vi "SetZeroFCG.vi"(8 "error in (no error)":errorcluster) -> (0 "error out":errorcluster)   [LabVIEW 2011]
uses:
  Variables/GlobalSetGetConfigureCamera.vi
  Variables/ccdChipPixels.vi
  Variables/GlobalSetGetHeidenhainParameters.vi
  Variables/GlobalSetNumberOfDigits_PhysikalInstruments.vi
  Variables/GrapRoi.vi
  Variables/GlobalGetPhysikalInstrumentsOnOff.vi
  Variables/StartStopMesaurement.vi
  Variables/GlobalGetMesaurementStatus.vi
  Variables/GlobalLaserEmissionOnOffInterlook.vi
  Variables/GlobalGetHeidenhainDriftOnOff.vi
  Variables/GlobalGetConfigurationStatus.vi
  Variables/GlobalGetInitialisationStatus.vi
  Variables/GlobalGetKoherasLaserOnOff.vi
  Variables/GlobalGetAOTFOnOff.vi
  Variables/GlobalGetAvantesSpectrometerOnOff.vi
  Variables/GlobalGetCamerasOnOff.vi
  Variables/SetRoi.vi
  Variables/GetPicture.vi
  Variables/StopGetPic.vi
  Variables/GlobalSetGetParametersAvantes.vi
  Variables/GlobalSetGetPositionParameters.vi
  Variables/GlobalSetGetTriggerForPointMeasurement.vi
  Variables/GlobalSetGetPixelOfRoi.vi
  Variables/GetSetGlobalPath2StoreStackData.vi
  Variables/cameraHandler.vi
  Variables/GlobalCameraDebugTemperature.vi
  Variables/ScannerMirrorStatus.vi
  Variables/GlobalGetSetMeasurementType.vi
  Variables/GlobalSetNumberOfDigits_Scanners.vi
  Variables/GlobalImage.vi
panel:
  in  "out":T1
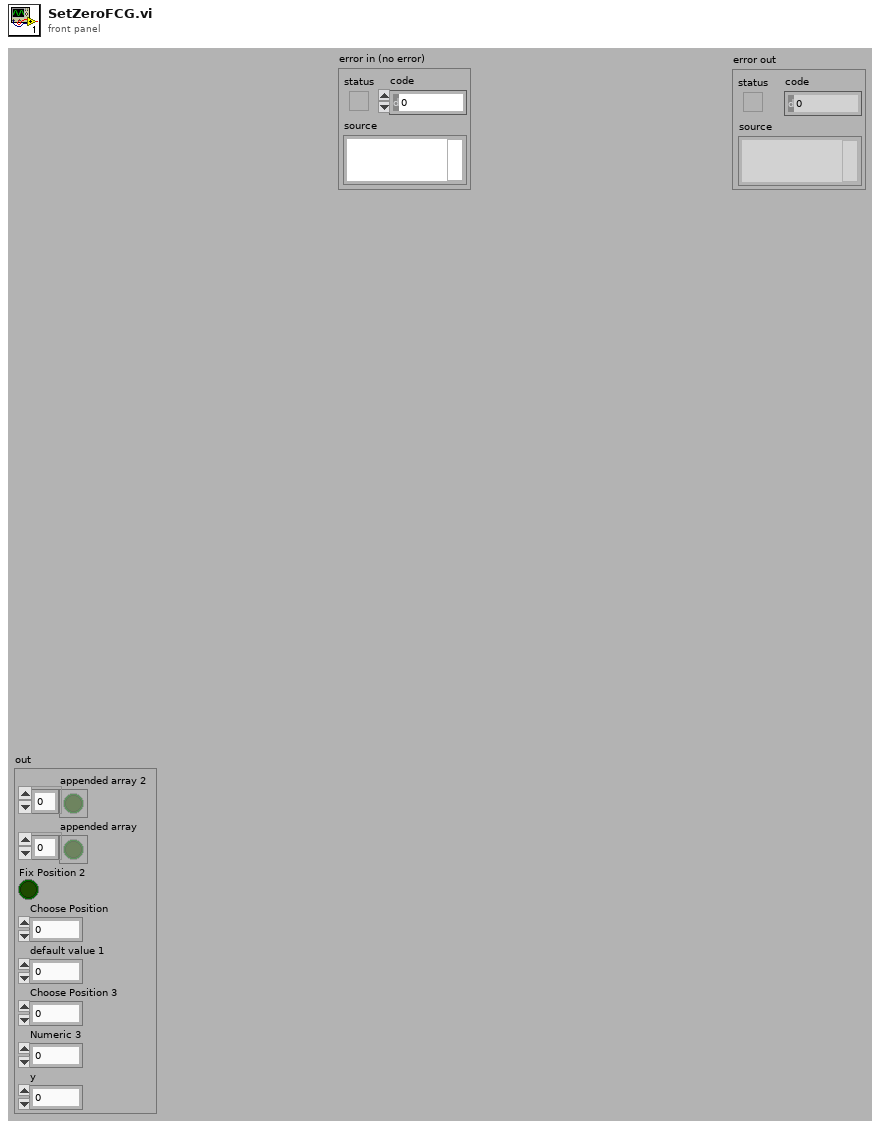
[diagram p1: front panel]
types:
  T1 = cluster{"appended array 2":bool[], "appended array":bool[], "Fix Position 2":bool, "Choose Position":dbl, "default value 1":dbl, "Choose Position 3":dbl, "Numeric 3":i32, "y":i32}
  T2 = cluster{"numbers of \nmeasurements":i16, "startPixel":u16, "stopPixel":u16, "intTime / [ms]":sgl, "backgroundSubtract":bool, "numAvg":u32}
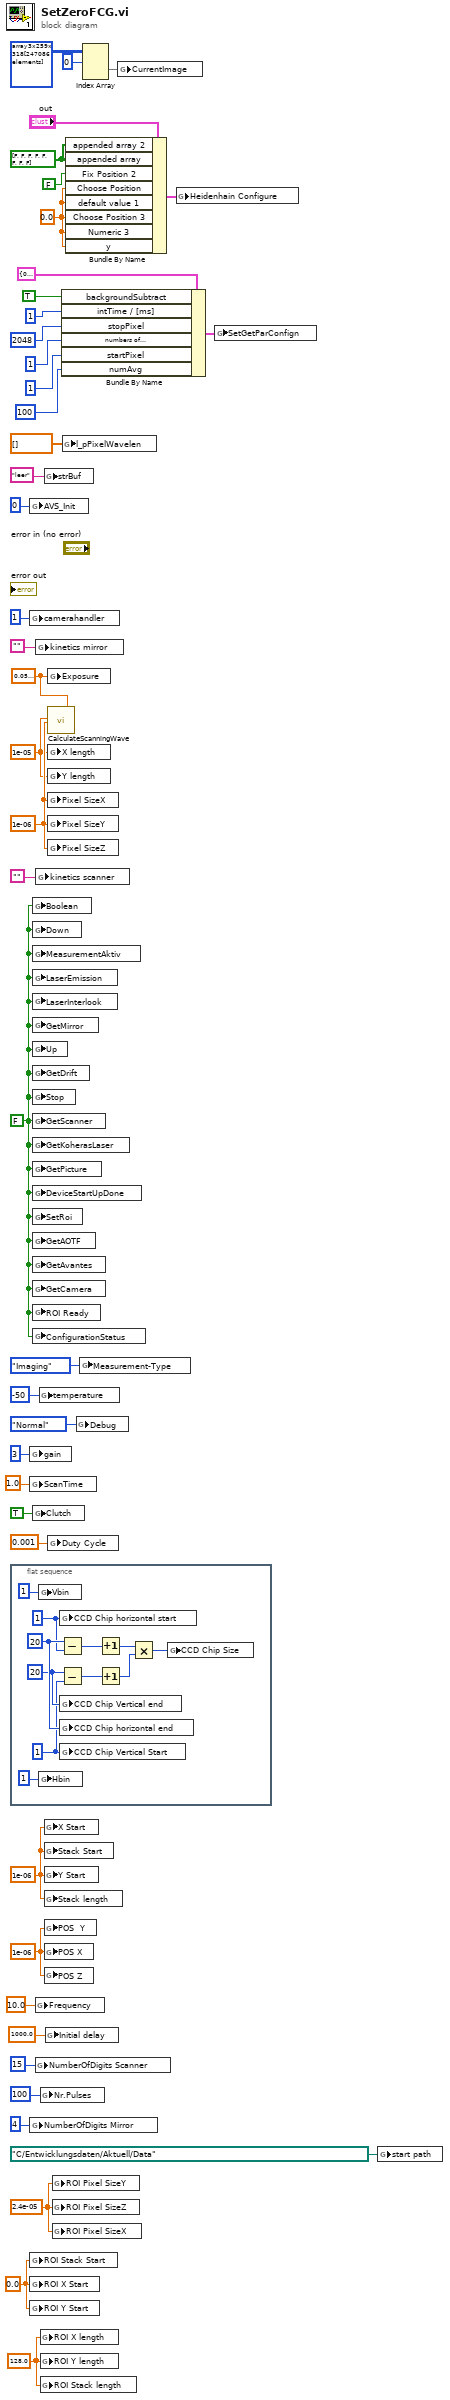
[diagram p0: block diagram]
diagram:
  w18 = 128.0 ("ROI Stack length")
  w19 = 0.0 ("ROI Stack Start")
  w20 = 2.4e-05 ("ROI Pixel SizeX")
  w14 = 1e-05 ("X length")
  w17 = 1e-06 ("X Start")
  w15 = 1e-06 ("Pixel SizeX")
  w29 = 1e-06 ("Duty Cycle")
  w1 = FALSE ("andor 2")
  w16 = sgl 0.05 ("ExpTime")
  w42 = 0.0 ("Choose Position")
  w43 = bool[] [FALSE, FALSE, FALSE, FALSE, FALSE, FALSE, FALSE, FALSE] ("appended array")
  n1 = flat-sequence {
    frame #0 {
      w48 = 20 ("CCD Chip Vertical end")
      w46 = 1 ("CCD Chip Vertical Start")
      w47 = 20 ("CCD Chip horizontal end")
      w45 = 1
      n2 = global write "GlobalSetGetConfigureCamera.vi" "Vbin"(1 ("Vbin")) -> ()
      n3 = global write "GlobalSetGetConfigureCamera.vi" "Hbin"(1 ("Hbin")) -> ()
      n4 = Subtract(x=w48, y=w45) -> (x-y=w50:i32)
      n5 = Subtract(x=w47, y=w46) -> (x-y=w49:i32)
      n6 = global write "ccdChipPixels.vi" "CCD Chip horizontal start"(w45) -> ()
      n7 = global write "ccdChipPixels.vi" "CCD Chip Vertical end"(w47) -> ()
      n8 = global write "ccdChipPixels.vi" "CCD Chip horizontal end"(w48) -> ()
      n9 = global write "ccdChipPixels.vi" "CCD Chip Vertical Start"(w46) -> ()
      n10 = Increment(x=w50) -> (x+1=w52:i32)
      n11 = Increment(x=w49) -> (x+1=w51:i32)
      n12 = Multiply(x=w52, y=w51) -> (x*y=w55:i32)
      n13 = global write "ccdChipPixels.vi" "CCD Chip Size"(w55) -> ()
    }
  }
  n14 = global write "GlobalSetGetParametersAvantes.vi" "AVS_Init"(0 ("AVS_Init")) -> ()
  n15 = global write "cameraHandler.vi" "camerahandler"(1 ("camerahandler")) -> ()
  n16 = global write "GlobalSetGetConfigureCamera.vi" "gain"(3 ("gain")) -> ()
  n17 = global write "GlobalSetGetPositionParameters.vi" "ScanTime"(1.0 ("Duty Cycle")) -> ()
  n18 = global write "GlobalSetNumberOfDigits_PhysikalInstruments.vi" "NumberOfDigits Mirror"(4 ("NumberOfDigits")) -> ()
  n19 = global write "GlobalSetGetPixelOfRoi.vi" "ROI Stack Start"(w19) -> ()
  n20 = global write "GlobalSetGetPixelOfRoi.vi" "ROI X Start"(w19) -> ()
  n21 = global write "GlobalSetGetPixelOfRoi.vi" "ROI Y Start"(w19) -> ()
  n22 = global write "StartStopMesaurement.vi" "Boolean"(w1) -> ()
  n23 = global write "GlobalSetGetHeidenhainParameters.vi" "Down"(w1) -> ()
  n24 = global write "GlobalGetMesaurementStatus.vi" "MeasurementAktiv"(w1) -> ()
  n25 = global write "GlobalLaserEmissionOnOffInterlook.vi" "LaserEmission"(w1) -> ()
  n26 = global write "GlobalLaserEmissionOnOffInterlook.vi" "LaserInterlook"(w1) -> ()
  n27 = global write "GlobalGetPhysikalInstrumentsOnOff.vi" "GetMirror"(w1) -> ()
  n28 = global write "GlobalSetGetHeidenhainParameters.vi" "Up"(w1) -> ()
  n29 = global write "GlobalGetHeidenhainDriftOnOff.vi" "GetDrift"(w1) -> ()
  n30 = global write "StopGetPic.vi" "Stop"(w1) -> ()
  n31 = global write "GlobalGetPhysikalInstrumentsOnOff.vi" "GetScanner"(w1) -> ()
  n32 = global write "GlobalGetKoherasLaserOnOff.vi" "GetKoherasLaser"(w1) -> ()
  n33 = global write "GetPicture.vi" "GetPicture"(w1) -> ()
  n34 = global write "GlobalGetInitialisationStatus.vi" "DeviceStartUpDone"(w1) -> ()
  n35 = global write "SetRoi.vi" "SetRoi"(w1) -> ()
  n36 = global write "GlobalGetAOTFOnOff.vi" "GetAOTF"(w1) -> ()
  n37 = global write "GlobalGetAvantesSpectrometerOnOff.vi" "GetAvantes"(w1) -> ()
  n38 = global write "GlobalGetCamerasOnOff.vi" "GetCamera"(w1) -> ()
  n39 = global write "GrapRoi.vi" "ROI Ready"(w1) -> ()
  n40 = global write "GlobalGetConfigurationStatus.vi" "ConfigurationStatus"(w1) -> ()
  n41 = global write "GlobalSetGetHeidenhainParameters.vi" "Clutch"(TRUE ("Clutch")) -> ()
  n42 = global write "GlobalSetGetTriggerForPointMeasurement.vi" "Frequency"(10.0 ("Frequency")) -> ()
  n43 = global write "GlobalSetNumberOfDigits_Scanners.vi" "NumberOfDigits Scanner"(15 ("NumberOfDigits Scanner")) -> ()
  n44 = global write "ScannerMirrorStatus.vi" "kinetics mirror"("") -> ()
  n45 = global write "ScannerMirrorStatus.vi" "kinetics scanner"("") -> ()
  n46 = global write "GlobalCameraDebugTemperature.vi" "temperature"(-50 ("temperature")) -> ()
  n47 = global write "GlobalSetGetTriggerForPointMeasurement.vi" "Nr.Pulses"(100 ("Nr.Pulses")) -> ()
  n48 = global write "GlobalSetGetPixelOfRoi.vi" "ROI X length"(w18) -> ()
  n49 = global write "GlobalSetGetPixelOfRoi.vi" "ROI Y length"(w18) -> ()
  n50 = global write "GlobalSetGetPixelOfRoi.vi" "ROI Stack length"(w18) -> ()
  n51 = global write "GlobalSetGetParametersAvantes.vi" "strBuf"("leer" ("strBuf")) -> ()
  n52 = global write "GlobalSetGetPixelOfRoi.vi" "X Start"(w17) -> ()
  n53 = global write "GlobalSetGetPixelOfRoi.vi" "Stack Start"(w17) -> ()
  n54 = global write "GlobalSetGetPixelOfRoi.vi" "Y Start"(w17) -> ()
  n55 = global write "GlobalSetGetPixelOfRoi.vi" "Stack length"(w17) -> ()
  n56 = global write "GlobalSetGetPositionParameters.vi" "POS  Y"(w29) -> ()
  n57 = global write "GlobalSetGetPositionParameters.vi" "POS X"(w29) -> ()
  n58 = global write "GlobalSetGetPositionParameters.vi" "POS Z"(w29) -> ()
  n59 = global write "GlobalSetGetTriggerForPointMeasurement.vi" "Initial delay"(1000.0 ("Initial delay")) -> ()
  n60 = global write "GlobalSetGetConfigureCamera.vi" "Exposure"(w16) -> ()
  n61 = call "CalculateScanningWave.vi"("X-length 3"=w14, "X-Delta 3"=w15, "kineticexposure"=w16) -> ()  [unwired: 14 in, 3 out]
  n62 = global write "GlobalSetGetPixelOfRoi.vi" "X length"(w14) -> ()
  n63 = global write "GlobalSetGetPixelOfRoi.vi" "Y length"(w14) -> ()
  n64 = global write "GlobalSetGetPixelOfRoi.vi" "Pixel SizeX"(w15) -> ()
  n65 = global write "GlobalSetGetPixelOfRoi.vi" "Pixel SizeY"(w15) -> ()
  n66 = global write "GlobalSetGetPixelOfRoi.vi" "Pixel SizeZ"(w15) -> ()
  n67 = global write "GlobalSetGetTriggerForPointMeasurement.vi" "Duty Cycle"(0.001 ("Duty Cycle")) -> ()
  n68 = global write "GlobalSetGetPixelOfRoi.vi" "ROI Pixel SizeY"(w20) -> ()
  n69 = global write "GlobalSetGetPixelOfRoi.vi" "ROI Pixel SizeZ"(w20) -> ()
  n70 = global write "GlobalSetGetPixelOfRoi.vi" "ROI Pixel SizeX"(w20) -> ()
  n71 = Bundle By Name(cluster=T2 {"numbers of \nmeasurements"=0, "startPixel"=0, "stopPixel"=0, "intTime / [ms]"=0.0, "backgroundSubtract"=FALSE, "numAvg"=0} ("out"), "backgroundSubtract"=TRUE, "intTime / [ms]"=u16 1 ("startPixel"), "stopPixel"=u16 2048, "numbers of \nmeasurements"=i16 1 ("numbers of \nmeasurements"), "startPixel"=u16 1, "numAvg"=u32 100) -> (w26:T2)
  n72 = global write "GlobalSetGetParametersAvantes.vi" "l_pPixelWavelen"(dbl[] [] ("l_pPixelWavelen")) -> ()
  n73 = Bundle By Name(cluster="out", "appended array 2"=w43, "appended array"=w43, "Fix Position 2"=FALSE, "Choose Position"=w42, "default value 1"=w42, "Choose Position 3"=w42, "Numeric 3"=w42, "y"=w42) -> (w27:T1)
  n74 = global write "GlobalCameraDebugTemperature.vi" "Debug"(enum16{"Debug", "Normal"}."Normal" ("Debug")) -> ()
  n75 = global write "GlobalGetSetMeasurementType.vi" "Measurement-Type"(enum32{"Diffusion", "Imaging"}."Imaging" ("Measurement-Type")) -> ()
  n76 = Index Array(array=i32[][][] array3x259x318[247086 elements] ("Array 2"), index (dim 0)=0 ("index (page)")) -> (element=w2:i32[][])  [unwired: 2 in]
  n77 = global write "GlobalImage.vi" "CurrentImage"(w2) -> ()
  n78 = global write "GlobalSetGetHeidenhainParameters.vi" "Heidenhain Configure"(w27) -> ()
  n79 = global write "GlobalSetGetParametersAvantes.vi" "SetGetParConfign"(w26) -> ()
  n80 = global write "GetSetGlobalPath2StoreStackData.vi" "start path"(path "C:/Entwicklungsdaten/Aktuell/Data" ("start path")) -> ()
